vi "Add to Created Files.vi"(8 "error in (no error)":errorcluster, 9 "Path to Replace (\"\")":path, 10 "Path to Add":path, 11 "QControl Creation in":refnum<class "QControl Creation.lvclass">) -> (3 "QControl Creation out":refnum<class "QControl Creation.lvclass">)   [LabVIEW 2015, in "QControl Creation.lvclass"]
doc: "<b> </b> <b> </b>\n©2016 Q Software Innovations, LLC (QSI)\nwritten by Quentin Alldredge\nproduced in LabVIEW 2015\n\nsupport@qsoftwareinnovations.com\nwww.qsoftwareinnovations.com\n\nAll rights reserved.\n\nRedistribution and use in source and binary forms, with or without modification, are permitted provided that the following conditions are met:\n\n * Redistributions of source code must retain the above copyright notice, this list of conditions and the following disclaimer.\n * Redistributions in binary form must reproduce the above copyright notice, this list of conditions and the following disclaimer in the documentation and/or other materials provided with the distribution.\n * Neither the name of Q Software Innovations, LLC. nor the names of its contributors may be used to endorse or promote products derived from this software without specific prior written permission.\n\nTHIS SOFTWARE IS PROVIDED BY THE COPYRIGHT HOLDERS AND CONTRIBUTORS \"AS IS\" AND ANY EXPRESS OR IMPLIED WARRANTIES, INCLUDING, BUT NOT LIMITED TO, THE IMPLIED WARRANTIES OF MERCHANTABILITY AND FITNESS FOR A PARTICULAR PURPOSE ARE DISCLAIMED. IN NO EVENT SHALL THE COPYRIGHT OWNER OR CONTRIBUTORS BE LIABLE FOR ANY DIRECT, INDIRECT, INCIDENTAL, SPECIAL, EXEMPLARY, OR CONSEQUENTIAL DAMAGES (INCLUDING, BUT NOT LIMITED TO, PROCUREMENT OF SUBSTITUTE GOODS OR SERVICES; LOSS OF USE, DATA, OR PROFITS; OR BUSINESS INTERRUPTION) HOWEVER CAUSED AND ON ANY THEORY OF LIABILITY, WHETHER IN CONTRACT, STRICT LIABILITY, OR TORT (INCLUDING NEGLIGENCE OR OTHERWISE) ARISING IN ANY WAY OUT OF THE USE OF THIS SOFTWARE, EVEN IF ADVISED OF THE POSSIBILITY OF SUCH DAMAGE."
uses:
  QControl Creation.lvclass
  QControl Creation.lvclass/QControl Creation.ctl
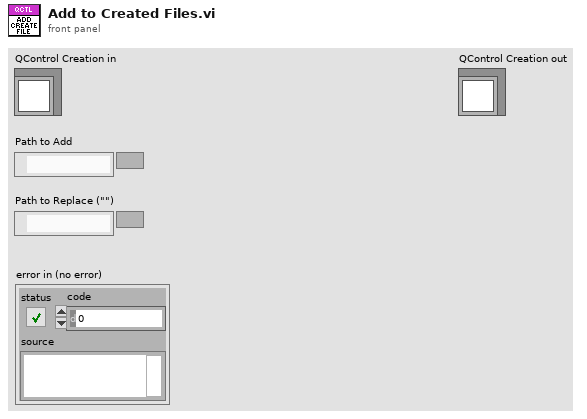
[diagram p1: front panel]
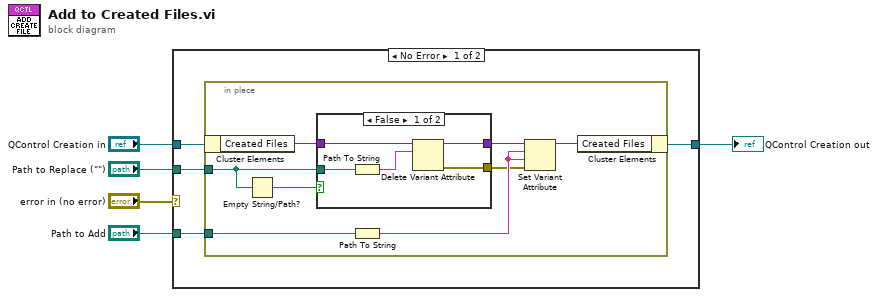
[diagram p0: block diagram]
diagram:
  n1 = case shown="No Error" "error in (no error)" {
    tunnel: "QControl Creation in" -> [w9 w24]
    tunnel: "Path to Add" -> [w8 _]
    tunnel: [w7 w24] -> w3
    tunnel: "Path to Replace (\"\")" -> [w6 _]
    frame No Error {
      n2 = in-place {
        in-place-border: w8 -> [w14]
        in-place-border: w6 -> [w15]
        n3 = in-place-cluster #1(w9) -> ("Created Files"=w16:variant)
        n4 = Empty String/Path?(string/path=w15) -> (empty?=w17:bool)
        n5 = case shown="False" w17 {
          tunnel: w16 -> [w22 w23]
          tunnel: w15 -> [w20 _]
          tunnel: [w21 w23] -> w13
          tunnel: [w18 _] -> w10
          frame False {
            n6 = Path To String(path=w20) -> (string=w19:string)
            n7 = Delete Variant Attribute(6:w19, 7:w22) -> (0:w18:errorcluster, 3:w21:variant)  [unwired: 1 in, 1 out]
          }
          frame True {
          }
        }
        n8 = Path To String(path=w14) -> (string=w11:string)
        n9 = Set Variant Attribute(Variant=w13, name=w11, value=w11, error in=w10) -> (Variant out=w12:variant)  [unwired: 2 out]
        n10 = in-place-cluster #1("Created Files"=w12) -> (w7:refnum<class "QControl Creation.lvclass">)
      }
    }
    frame Error {
    }
  }
  "QControl Creation out" <- w3
